vi "Name Counter.vi"(0 "Input String":string, 1 "Remove Consonants?":bool) -> (2 "Consonant Count":dbl, 3 "Output":string, 4 "Vowel Count":dbl)   [LabVIEW 2017]
panel:
  out "Info Sentence":string
  out "Sentence":string
  in  "Name?":bool
  out "Without Vowels":string
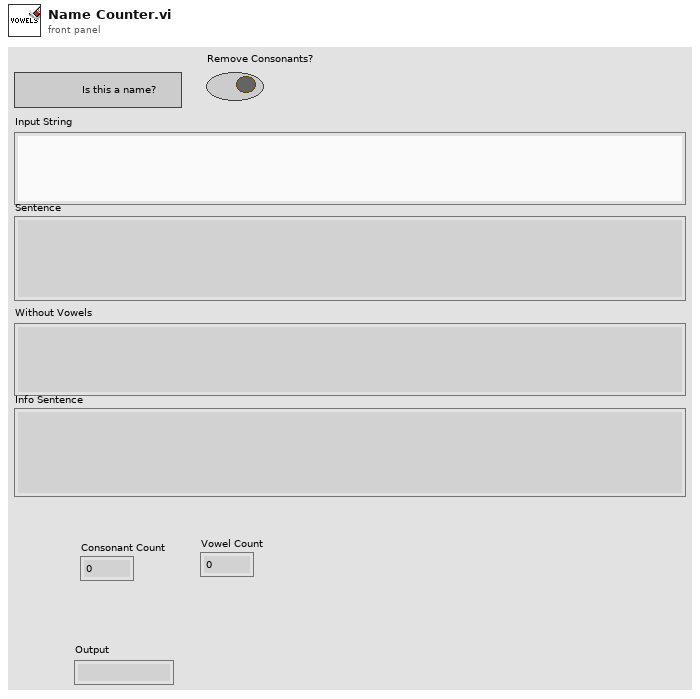
[diagram p1: front panel]
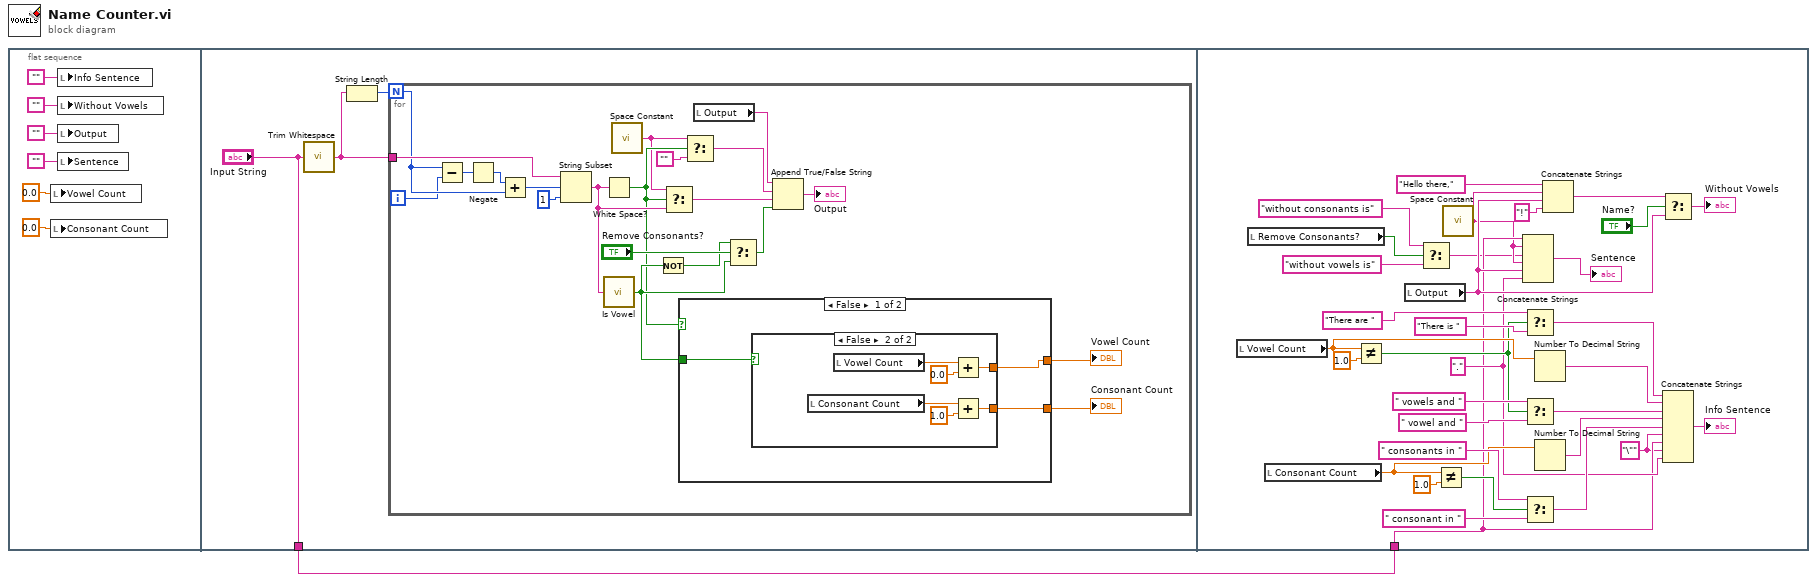
[diagram p0: block diagram]
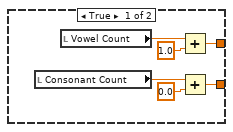
[diagram p2: hidden frame]
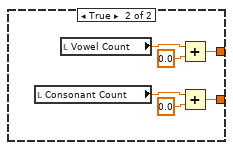
[diagram p3: hidden frame]
diagram:
  n1 = flat-sequence {
    tunnel: ["Input String"] -> w1
    tunnel: w1 -> [w59]
    frame #0 {
      n2 = local write "Vowel Count"(0.0 ("Vow Count")) -> ()
      n3 = local write "Consonant Count"(0.0 ("Con Count")) -> ()
      n4 = local write "Info Sentence"("") -> ()
      n5 = local write "Without Vowels"("") -> ()
      n6 = local write "Output"("") -> ()
      n7 = local write "Sentence"("") -> ()
    }
    frame #1 {
      n8 = call <vilib>:"Trim Whitespace.vi"("string"="Input String") -> ("trimmed string"=w9:string)  [unwired: 1 in]
      n9 = String Length(string=w9) -> (length=w10:i32)
      n10 = for {
        N: w10 -> [w26]
        tunnel: w9 -> [w31]
        i -> [w22]
        n11 = Subtract(x=w26, y=w22) -> (x-y=w28:i32)
        n12 = Negate(x=w28) -> (-x=w27:i32)
        n13 = Add(x=w27, y=w26) -> (x+y=w25:i32)
        n14 = String Subset(string=w31, offset (0)=w25, length (rest)=1 ("length (rest)")) -> (substring=w29:string)
        n15 = White Space?(1:w29) -> (0:w13:bool)
        n16 = call "Is Vowel.vi"("Single Character"=w29) -> ("Is Vowel?"=w17:bool)
        n17 = call <vilib>:"Space Constant.vi"() -> ("String"=w12:string)
        n18 = Not(x=w17) -> (.not. x?=w16:bool)
        n19 = Select(t=w12, s=w13, f=w29) -> (s? t:f=w19:string)
        n20 = case shown="False" w13 {
          tunnel: [w34 w47] -> w24
          tunnel: [w33 w48] -> w23
          tunnel: w17 -> [w32 _]
          frame False {
            n21 = case shown="False" w32 {
              tunnel: [w35 w41] -> w34
              tunnel: [w36 w42] -> w33
              frame True {
                n22 = local read "Consonant Count"() -> (w37:dbl)
                n23 = local read "Vowel Count"() -> (w40:dbl)
                n24 = Add(x=w40, y=1.0) -> (x+y=w36:dbl)
                n25 = Add(x=w37, y=0.0) -> (x+y=w35:dbl)
              }
              frame False {
                n26 = local read "Consonant Count"() -> (w43:dbl)
                n27 = local read "Vowel Count"() -> (w46:dbl)
                n28 = Add(x=w46, y=0.0) -> (x+y=w42:dbl)
                n29 = Add(x=w43, y=1.0) -> (x+y=w41:dbl)
              }
            }
          }
          frame True {
            n30 = local read "Consonant Count"() -> (w49:dbl)
            n31 = local read "Vowel Count"() -> (w52:dbl)
            n32 = Add(x=w52, y=0.0) -> (x+y=w48:dbl)
            n33 = Add(x=w49, y=0.0) -> (x+y=w47:dbl)
          }
        }
        "Consonant Count" <- w24
        "Vowel Count" <- w23
        n34 = Select(t=w12, s=w13, f="") -> (s? t:f=w11:string)
        n35 = local read "Output"() -> (w20:string)
        n36 = Select(t=w16, s="Remove Consonants?", f=w17) -> (s? t:f=w15:bool)
        n37 = Append True/False String(1:w15, 2:w19, 3:w11, 4:w20) -> (0:→"Output":string)
      }
    }
    frame #2 {
      w58 = "\"" ("string")
      w60 = "." ("string")
      n38 = local read "Vowel Count"() -> (w72:dbl)
      n39 = local read "Remove Consonants?"() -> (w54:bool)
      n40 = local read "Consonant Count"() -> (w66:dbl)
      n41 = Not Equal?(x=w72, y=1.0) -> (x != y?=w61:bool)
      n42 = local read "Output"() -> (w81:string)
      n43 = Select(t="without consonants is", s=w54, f="without vowels is" ("string")) -> (s? t:f=w55:string)
      n44 = Not Equal?(x=w66, y=1.0) -> (x != y?=w67:bool)
      n45 = call <vilib>:"Space Constant.vi"() -> ("String"=w57:string)
      n46 = Concatenate Strings(w59, w57, w55, w57, w81, w60) -> (→"Sentence":string)
      n47 = Select(t="There are " ("string"), s=w61, f="There is " ("string")) -> (s? t:f=w64:string)
      n48 = Select(t=" vowels and " ("string"), s=w61, f=" vowel and " ("string")) -> (s? t:f=w74:string)
      n49 = Select(t=" consonants in " ("string"), s=w67, f=" consonant in " ("string")) -> (s? t:f=w69:string)
      n50 = Number To Decimal String(number=w72) -> (decimal integer string=w79:string)  [unwired: 1 in]
      n51 = Number To Decimal String(number=w66) -> (decimal integer string=w78:string)  [unwired: 1 in]
      n52 = Concatenate Strings("Hello there," ("string"), w57, w81, "!" ("string")) -> (w84:string)
      n53 = Select(t=w84, s="Name?", f=w81) -> (s? t:f=→"Without Vowels":string)
      n54 = Concatenate Strings(w64, w79, w74, w78, w69, w58, w59, w58, w60) -> (→"Info Sentence":string)
    }
  }
